vi "Brass Logging Tool.vi"(0 "GEA2 Reference In":refnum<k24>, 5 "Standalone?":bool=TRUE, 7 "Board Index":i32, 11 "Error In":errorcluster) -> (4 "GEA2 Reference Out":refnum<k24>, 6 "Brass Logging":T1={"Basket speed"=0, "Shaft Speed"=0, "Folding"=0, "Jerk"=0, "Jerk Delta"=0, "State"="Unknown", "Counter"=0, "Motor Current"=0.0}, 15 "Error Out":errorcluster)   [LabVIEW 2016]
uses:
  Q:/Common/DLLs/GEA3/GeaCommunication.dll
  Common/DLLs/GEA3/GeaCommunication.dll
  Common/LabVIEW GEA2 Toolkit/LabVIEW_GEA2_Toolkit.lvlibp/type defs/Data Out.ctl
  type defs/Brass_Logging.ctl
  Common/LabVIEW GEA2 Toolkit/LabVIEW_GEA2_Toolkit.lvlibp/type defs/Source_Destination.ctl
  Common/LabVIEW GEA2 Toolkit/LabVIEW_GEA2_Toolkit.lvlibp/type defs/ERD Write Data In.ctl
  Common/LabVIEW GEA2 Toolkit/LabVIEW_GEA2_Toolkit.lvlibp/type defs/Data Type.ctl
  Common/LabVIEW GEA2 Toolkit/LabVIEW_GEA2_Toolkit.lvlibp
panel:
  in  "Stop logging":bool
  in  "Brass Logging":T1={"Basket speed"=0, "Shaft Speed"=0, "Folding"=0, "Jerk"=0, "Jerk Delta"=0, "State"="Accel", "Counter"=0, "Motor Current"=0.0}
  out "Coverted Data Out":T2 {"CRC" format="%04x"; "Length" format="%02x"; "Command" format="%02x"; "Destination" format="%02x"; "Source" format="%02x"}
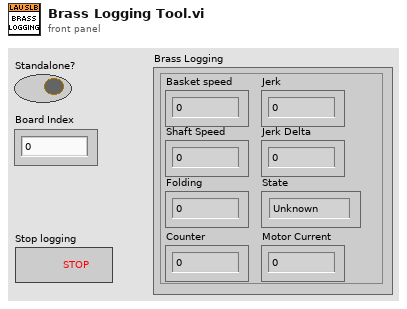
[diagram p1: front panel]
types:
  T1 = typedef "Brass_Logging.ctl" = cluster{"Basket speed":u16, "Shaft Speed":u16, "Folding":i32, "Jerk":i32, "Jerk Delta":u32, "State":string, "Counter":u8, "Motor Current":dbl}
  T2 = typedef "LabVIEW_GEA2_Toolkit.lvlibp/Data Out.ctl" = cluster{"Source":u8, "Destination":u8, "Command":u8, "Length":u8, "CRC":u16, "Message":string}
  T3 = typedef "LabVIEW_GEA2_Toolkit.lvlibp/ERD Write Data In.ctl" = cluster{"ERD Number":u16, "Data Type":T4, "Data":string}
  T4 = typedef "LabVIEW_GEA2_Toolkit.lvlibp/Data Type.ctl" = enum16{"string", "boolean", "uint8_t", "uint16_t", "uint32_t", "uint64_t", "int8_t", "int16_t", "int32_t", "int64_t"}
  T5 = typedef "LabVIEW_GEA2_Toolkit.lvlibp/Source_Destination.ctl" = cluster{"Source":u8, "Destination":u8}
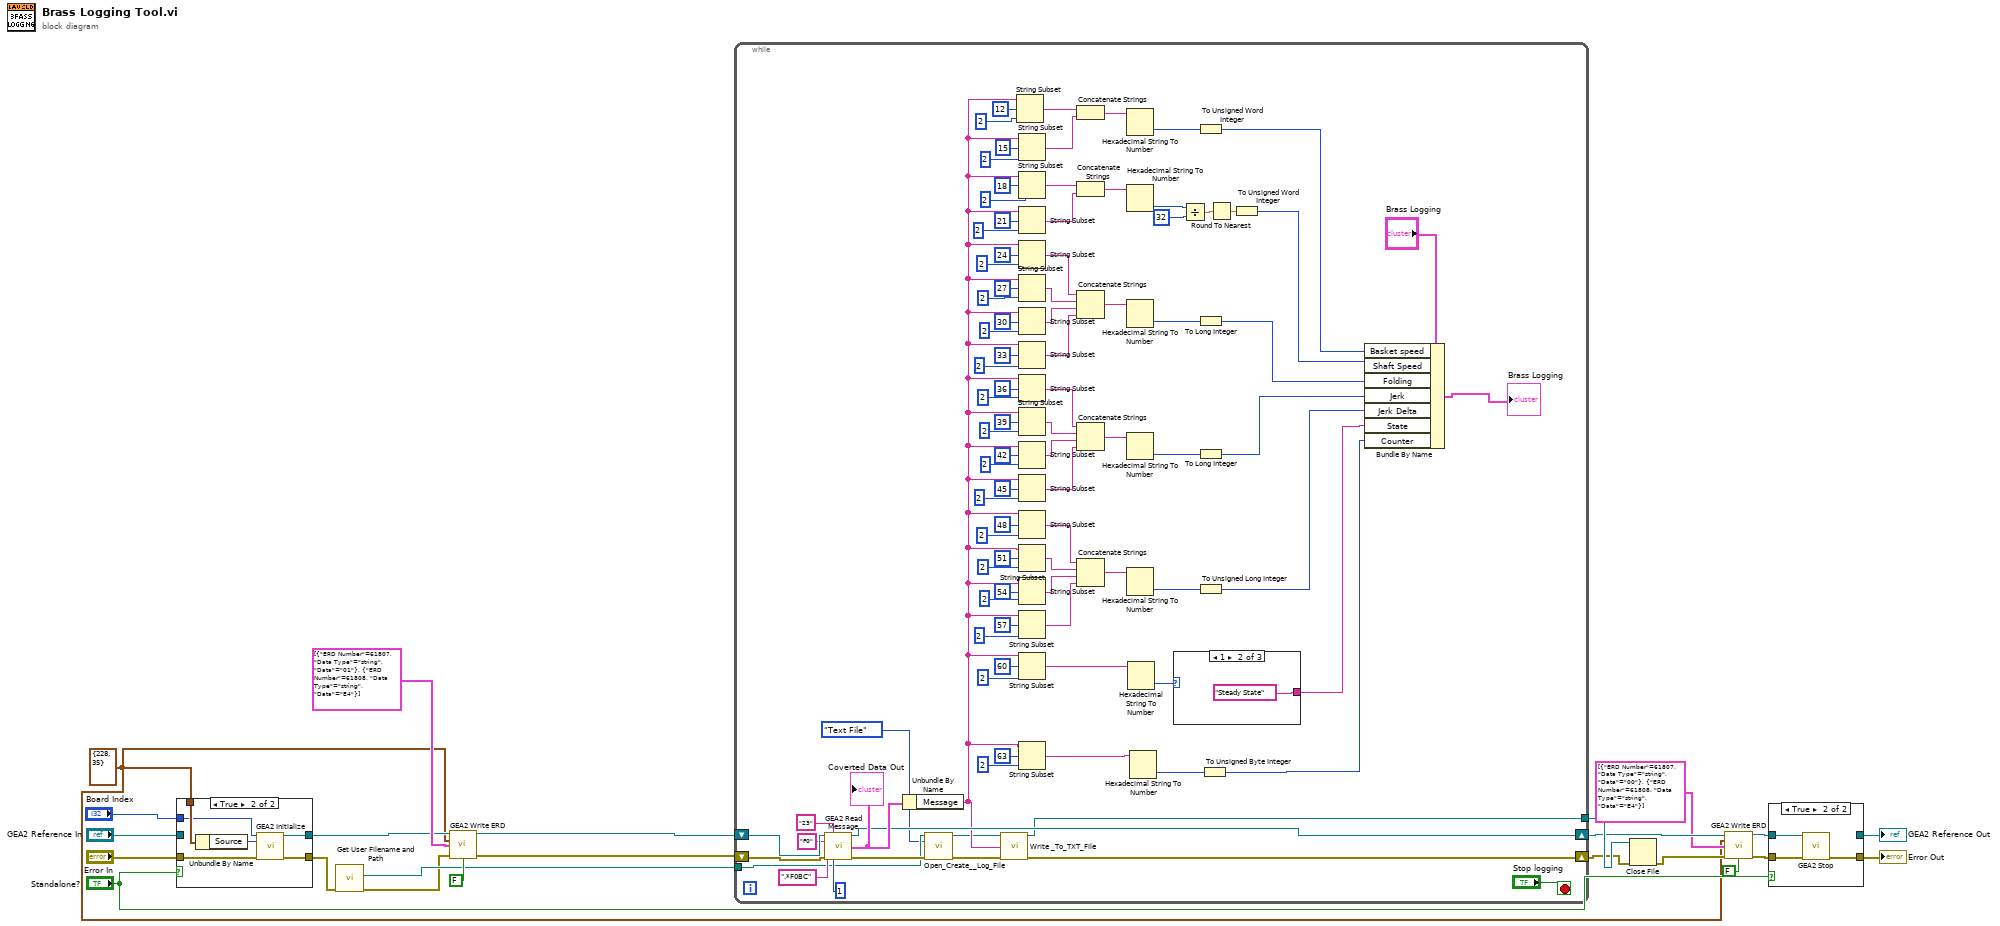
[diagram p0: block diagram]
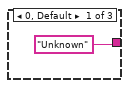
[diagram p2: hidden frame]
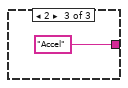
[diagram p3: hidden frame]
diagram:
  w3 = T5 {"Source"=228, "Destination"=35} ("GEA Inputs")
  n1 = case shown="True" "Standalone?" {
    tunnel: "Error In" -> [w24 w31]
    tunnel: [w24 w30] -> w17
    tunnel: "GEA2 Reference In" -> [w25 _]
    tunnel: [w25 w29] -> w13
    tunnel: w3 -> [_ w27]
    tunnel: "Board Index" -> [_ w26]
    frame False {
    }
    frame True {
      n2 = Unbundle By Name(w27) -> ("Source"=w28:u8)
      n3 = call "GEA2 Initialize.vi"("Board Index"=w26, "Source Address"=w28, "error in"=w31) -> ("GEA2 Reference Out"=w29:refnum<k24>, "error out"=w30:errorcluster)  [unwired: 10 in, 1 out]
    }
  }
  n4 = call "Get User Filename and Path.vi"("error in (no error)"=w17) -> ("error out"=w1:errorcluster, "TXT File Path"=w2:path)  [unwired: 8 in, 1 out]
  n5 = call "GEA2 Write ERD.vi"("GEA2 Reference In"=w13, "GEA Inputs"=w3, "Write ERD List"=T3[] [{"ERD Number"=61807, "Data Type"=enum."string", "Data"="01"}, {"ERD Number"=61808, "Data Type"=enum."string", "Data"="E4"}], "Error In"=w1, "Verify ERD Response?"=FALSE) -> ("GEA2 Reference Out"=w11:refnum<k24>, "Error Out"=w12:errorcluster)  [unwired: 8 in, 1 out]
  n6 = while {
    shift-right: [w40] -> w9
    shift-left: w11 -> [w126]
    shift-right: [w38] -> w15
    shift-left: w12 -> [w125]
    tunnel: w2 -> [w34]
    tunnel: [w37] -> w16
    stop <- "Stop logging" stop-if-true
    n7 = call "GEA2 Read Message.vi"("GEA2 Reference In"=w126, "Expected Source"="23", "Expected Command"="F0", "Expected Data"=".*F0BC", "Error In"=w125, "# of Tries"=u8 1) -> ("GEA2 Reference Out"=w40:refnum<k24>, "Coverted Data Out"=w41:T2, "Error Out"=w35:errorcluster)  [unwired: 6 in, 1 out]
    "Coverted Data Out" <- w41
    n8 = Unbundle By Name(w41) -> ("Message"=w39:string)
    n9 = call "Open_Create__Log_File.vi"("File Path Control"=w34, "Enum"=enum16{"CSV File", "Text File"}."Text File", "Error In"=w35) -> ("refnum out"=w32:refnum<file>, "Error Out"=w36:errorcluster)  [unwired: 10 in, 1 out]
    n10 = call "Write _To_TXT_File.vi"("refnum"=w32, "text"=w39, "error in"=w36) -> ("refnum out"=w37:refnum<file>, "error out"=w38:errorcluster)  [unwired: 10 in, 1 out]
    n11 = String Subset(string=w39, offset (0)=12, length (rest)=2 ("length (rest)")) -> (substring=w116:string)
    n12 = String Subset(string=w39, offset (0)=15, length (rest)=2 ("length (rest)")) -> (substring=w115:string)
    n13 = String Subset(string=w39, offset (0)=18, length (rest)=2 ("length (rest)")) -> (substring=w110:string)
    n14 = String Subset(string=w39, offset (0)=21, length (rest)=2 ("length (rest)")) -> (substring=w109:string)
    n15 = String Subset(string=w39, offset (0)=24, length (rest)=2 ("length (rest)")) -> (substring=w100:string)
    n16 = String Subset(string=w39, offset (0)=27, length (rest)=2 ("length (rest)")) -> (substring=w99:string)
    n17 = String Subset(string=w39, offset (0)=30, length (rest)=2 ("length (rest)")) -> (substring=w98:string)
    n18 = String Subset(string=w39, offset (0)=33, length (rest)=2 ("length (rest)")) -> (substring=w97:string)
    n19 = String Subset(string=w39, offset (0)=36, length (rest)=2 ("length (rest)")) -> (substring=w88:string)
    n20 = String Subset(string=w39, offset (0)=39, length (rest)=2 ("length (rest)")) -> (substring=w87:string)
    n21 = String Subset(string=w39, offset (0)=42, length (rest)=2 ("length (rest)")) -> (substring=w86:string)
    n22 = String Subset(string=w39, offset (0)=45, length (rest)=2 ("length (rest)")) -> (substring=w85:string)
    n23 = String Subset(string=w39, offset (0)=48, length (rest)=2 ("length (rest)")) -> (substring=w76:string)
    n24 = String Subset(string=w39, offset (0)=51, length (rest)=2 ("length (rest)")) -> (substring=w75:string)
    n25 = String Subset(string=w39, offset (0)=54, length (rest)=2 ("length (rest)")) -> (substring=w74:string)
    n26 = String Subset(string=w39, offset (0)=57, length (rest)=2 ("length (rest)")) -> (substring=w73:string)
    n27 = String Subset(string=w39, offset (0)=60, length (rest)=2 ("length (rest)")) -> (substring=w63:string)
    n28 = String Subset(string=w39, offset (0)=63, length (rest)=2 ("length (rest)")) -> (substring=w61:string)
    n29 = Concatenate Strings(w116, w115) -> (w68:string)
    n30 = Concatenate Strings(w110, w109) -> (w67:string)
    n31 = Concatenate Strings(w100, w99, w98, w97) -> (w66:string)
    n32 = Concatenate Strings(w88, w87, w86, w85) -> (w65:string)
    n33 = Concatenate Strings(w76, w75, w74, w73) -> (w64:string)
    n34 = Hexadecimal String To Number(string=w68) -> (number=w60:u32)  [unwired: 2 in, 1 out]
    n35 = Hexadecimal String To Number(string=w67) -> (number=w55:u32)  [unwired: 2 in, 1 out]
    n36 = Hexadecimal String To Number(string=w66) -> (number=w59:u32)  [unwired: 2 in, 1 out]
    n37 = Hexadecimal String To Number(string=w65) -> (number=w58:u32)  [unwired: 2 in, 1 out]
    n38 = Hexadecimal String To Number(string=w64) -> (number=w57:u32)  [unwired: 2 in, 1 out]
    n39 = Hexadecimal String To Number(string=w63) -> (number=w62:u32)  [unwired: 2 in, 1 out]
    n40 = Hexadecimal String To Number(string=w61) -> (number=w56:u32)  [unwired: 2 in, 1 out]
    n41 = case shown="1" w62 {
      tunnel: ["Unknown" "Steady State" "Accel"] -> w45
      frame 0, Default {
      }
      frame 1 {
      }
      frame 2 {
      }
    }
    n42 = Divide(x=w55, y=u32 32) -> (x/y=w53:dbl)
    n43 = To Unsigned Word Integer(number=w60) -> (unsigned 16bit integer=w50:u16)
    n44 = To Long Integer(number=w59) -> (32bit integer=w48:i32)
    n45 = To Long Integer(number=w58) -> (32bit integer=w47:i32)
    n46 = To Unsigned Long Integer(number=w57) -> (unsigned 32bit integer=w46:u32)
    n47 = To Unsigned Byte Integer(number=w56) -> (unsigned 8bit integer=w44:u8)
    n48 = Round To Nearest(number=w53) -> (nearest integer value=w52:dbl)
    n49 = To Unsigned Word Integer(number=w52) -> (unsigned 16bit integer=w49:u16)
    n50 = Bundle By Name(cluster="Brass Logging", "Basket speed"=w50, "Shaft Speed"=w49, "Folding"=w48, "Jerk"=w47, "Jerk Delta"=w46, "State"=w45, "Counter"=w44) -> (→"Brass Logging":T1)
  }
  n51 = Close File(refnum=w16, error in=w15) -> (error out=w7:errorcluster)  [unwired: 1 out]
  n52 = call "GEA2 Write ERD.vi"("GEA2 Reference In"=w9, "GEA Inputs"=w3, "Write ERD List"=T3[] [{"ERD Number"=61807, "Data Type"=enum."string", "Data"="00"}, {"ERD Number"=61808, "Data Type"=enum."string", "Data"="E4"}], "Error In"=w7, "Verify ERD Response?"=FALSE) -> ("GEA2 Reference Out"=w8:refnum<k24>, "Error Out"=w6:errorcluster)  [unwired: 8 in, 1 out]
  n53 = case shown="True" "Standalone?" {
    tunnel: [w131 w134] -> w20
    tunnel: w6 -> [w131 w133]
    tunnel: w8 -> [w130 w132]
    tunnel: [w130 _] -> w21
    frame False {
    }
    frame True {
      n54 = call "GEA2 Stop.vi"("GEA2 Reference In"=w132, "Error In"=w133) -> ("Error Out"=w134:errorcluster)  [unwired: 13 in]
    }
  }
  "GEA2 Reference Out" <- w21
  "Error Out" <- w20
